vi "ADCQueueDrivervi.vi"(0 "Queue Name":string, 5 "Enqueue State":T1, 7 "Array State":T1[](array[typedef]), 11 "error in":errorcluster, 13 "Queue Operations":T2) -> (4 "Dequeue State":T1, 15 "error out":errorcluster)   [LabVIEW 2023]
doc: "This is the simple queue driver which can enqueue and dequeue states into a queue and use it further."
uses:
  Type def/QueueOperations.ctl
  Type def/variant.ctl
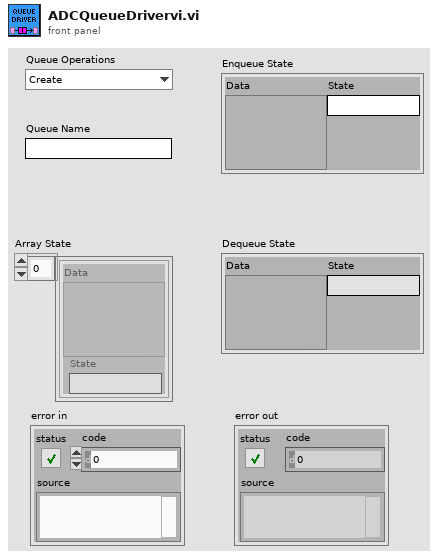
[diagram p1: front panel]
types:
  T1 = typedef "variant.ctl" = cluster{"Data":variant, "State":string}
  T2 = typedef "QueueOperations.ctl" = enum16{"Create", "Enqueue", "Enqueue N elements", "Dequeue", "Flush", "Release"}
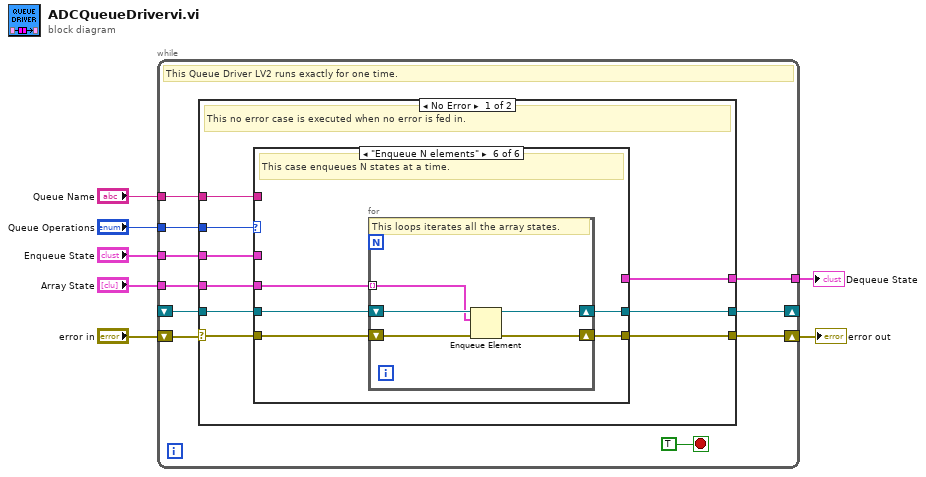
[diagram p0: block diagram]
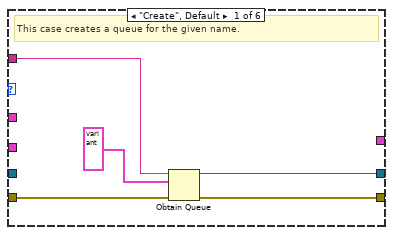
[diagram p2: hidden frame]
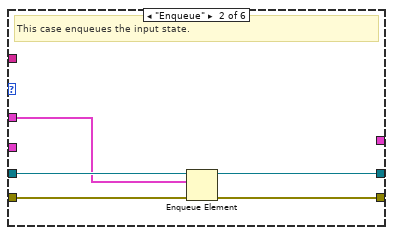
[diagram p3: hidden frame]
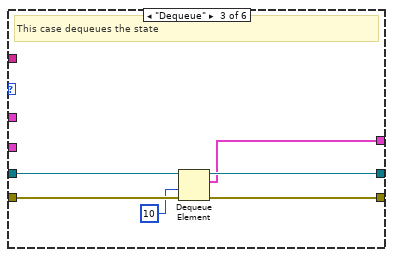
[diagram p4: hidden frame]
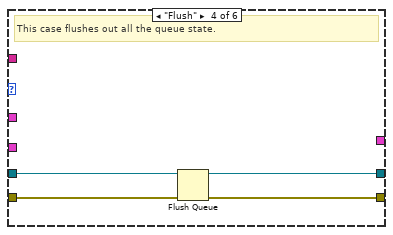
[diagram p5: hidden frame]
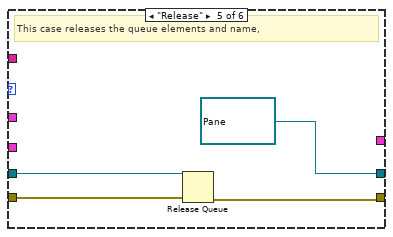
[diagram p6: hidden frame]
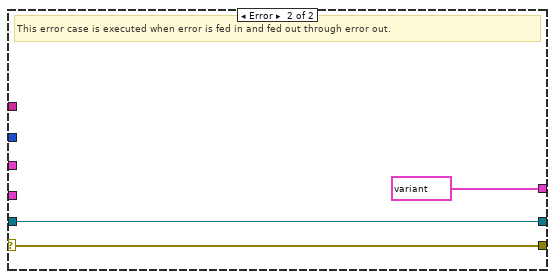
[diagram p7: hidden frame]
diagram:
  n1 = while {
    shift-right: [w15] -> w6
    shift-left: "error in" -> [w17]
    tunnel: "Queue Operations" -> [w16]
    tunnel: "Queue Name" -> [w14]
    tunnel: "Enqueue State" -> [w13]
    tunnel: [w11] -> w1
    shift-right: [w9] -> _
    shift-left: _ -> [w8]
    tunnel: "Array State" -> [w10]
    stop <- TRUE stop-if-true
    # "This Queue Driver LV2 runs exactly for one time."
    n2 = case shown="No Error" w17 {
      selector: w17 -> [w25 w63]
      tunnel: w16 -> [w26 _]
      tunnel: [w24 w63] -> w15
      tunnel: w14 -> [w23 _]
      tunnel: w13 -> [w22 _]
      tunnel: [w18 T1 {"Data"=variant, "State"="Error"}] -> w11
      tunnel: w10 -> [w21 _]
      tunnel: [w20 w62] -> w9
      tunnel: w8 -> [w19 w62]
      frame No Error {
        # "This no error case is executed when no error is fed in."
        n3 = case shown="\"Enqueue N elements\"" w26 {
          tunnel: w25 -> [w31 w36 w42 w46 w50 w55]
          tunnel: [w30 w35 w41 w45 w49 w54] -> w24
          tunnel: w23 -> [w29 _ _ _ _ _]
          tunnel: w22 -> [_ w32 _ _ _ _]
          tunnel: w21 -> [_ _ _ _ _ w53]
          tunnel: [w27 w33 w38 w43 refnum<queue> refnum ("queue out") w51] -> w20
          tunnel: w19 -> [_ w34 w39 w44 w48 w52]
          tunnel: [_ _ w37 _ _ _] -> w18
          frame "Create", Default {
            # "This case creates a queue for the given name."
            n4 = Obtain Queue(name (unnamed)=w29, element data type=T1 {"Data"=variant, "State"=""}, error in (no error)=w31) -> (queue out=w27:refnum<queue>, error out=w30:errorcluster)  [unwired: 2 in, 1 out]
          }
          frame "Enqueue" {
            # "This case enqueues the input state."
            n5 = Enqueue Element(queue=w34, element=w32, error in (no error)=w36) -> (queue out=w33:refnum<queue>, error out=w35:errorcluster)  [unwired: 1 in, 1 out]
          }
          frame "Dequeue" {
            # "This case dequeues the state"
            n6 = Dequeue Element(queue=w39, timeout in ms (-1)=10, error in (no error)=w42) -> (queue out=w38:refnum<queue>, element=w37:T1, error out=w41:errorcluster)  [unwired: 1 out]
          }
          frame "Flush" {
            # "This case flushes out all the queue state."
            n7 = Flush Queue(queue=w44, error in (no error)=w46) -> (queue out=w43:refnum<queue>, error out=w45:errorcluster)  [unwired: 1 out]
          }
          frame "Release" {
            # "This case releases the queue elements and name,"
            n8 = Release Queue(queue=w48, error in (no error)=w50) -> (error out=w49:errorcluster)  [unwired: 1 in, 2 out]
          }
          frame "Enqueue N elements" {
            # "This case enqueues N states at a time."
            n9 = for {
              shift-right: [w57] -> w51
              shift-left: w52 -> [w58]
              shift-right: [w59] -> w54
              shift-left: w55 -> [w60]
              tunnel: w53 -> [w56] mode=indexing
              # "This loops iterates all the array states."
              n10 = Enqueue Element(queue=w58, element=w56, error in (no error)=w60) -> (queue out=w57:refnum<queue>, error out=w59:errorcluster)  [unwired: 1 in, 1 out]
            }
          }
        }
      }
      frame Error {
        # "This error case is executed when error is fed in and fed out through error out."
      }
    }
  }
  "error out" <- w6
  "Dequeue State" <- w1
